vi "testFit.vi"() -> ()   [LabVIEW 2011]
uses:
  <vilib>/Analysis/NI_AALPro.lvlib
panel:
  out "XY Graph":cluster{"Value":dbl[], "Value":dbl[]}[](graph)
  out "Best Exponential Fit":dbl[](array[numeric])
  out "offset 2":dbl=nan
  out "damping":dbl=nan
  out "amplitude":dbl=nan
  in  "amp":dbl=100.0
  in  "alpha":dbl=-0.1
  in  "offset":dbl=20.0
  out "P array":dbl[](array[numeric])
  out "t array":dbl[](array[numeric])
  in  "dt":dbl=1.0
  in  "t":dbl
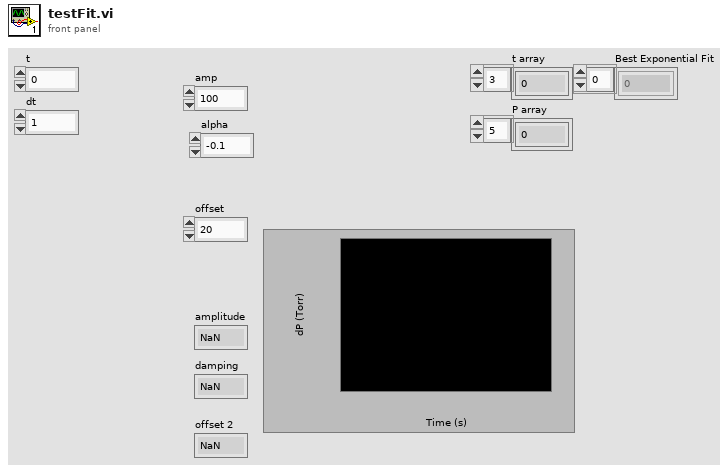
[diagram p1: front panel]
types:
  T1 = cluster{"amp min":dbl, "amp max":dbl, "damping min":dbl, "damping max":dbl, "offset min":dbl, "offset max":dbl}
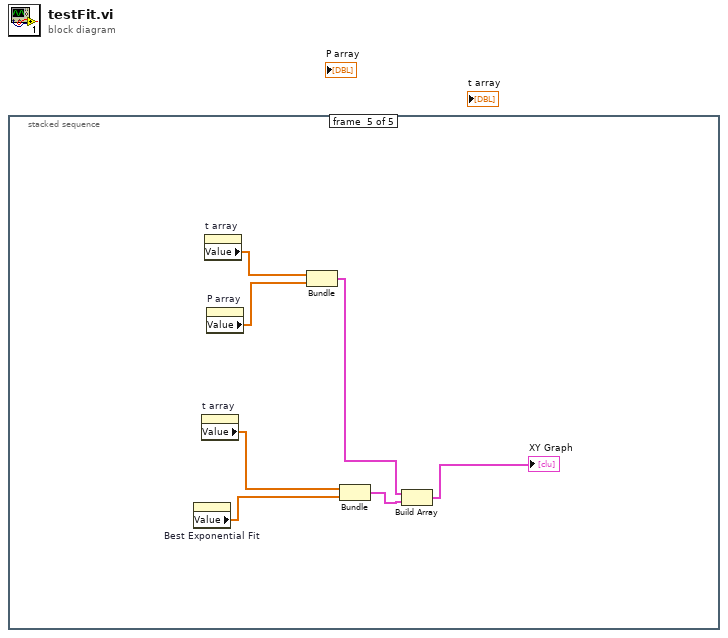
[diagram p0: block diagram]
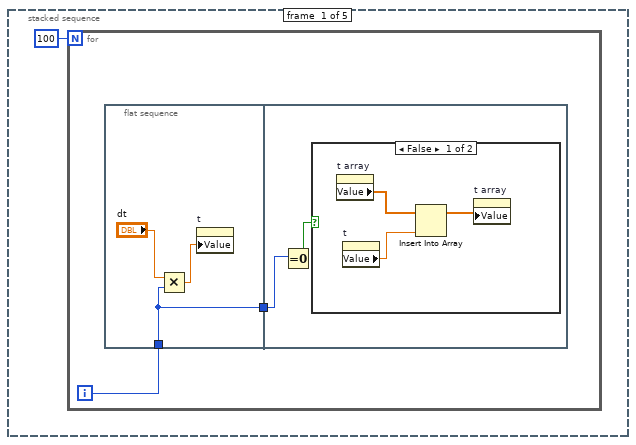
[diagram p2: hidden frame]
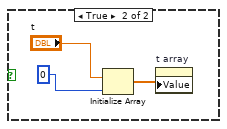
[diagram p3: hidden frame]
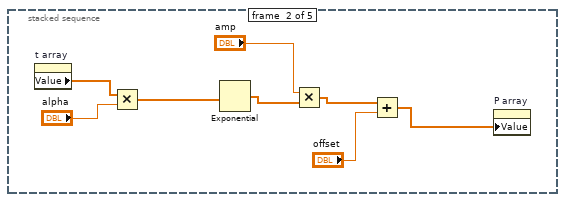
[diagram p4: hidden frame]
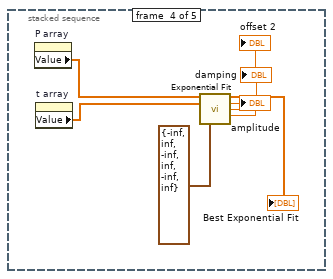
[diagram p6: hidden frame]
diagram:
  n1 = stacked-sequence {
    frame #0 {
      n2 = for {
        N: 100 -> [_]
        i -> [w3]
        n3 = flat-sequence {
          tunnel: w3 -> [w4]
          tunnel: [w4] -> w2
          tunnel: w2 -> [w8]
          frame #0 {
            n4 = Multiply(x="dt", y=w4) -> (x*y=w5:dbl)
            n5 = property on="t" class="DigNum (strict)"("Value"=w5) -> ()  [unwired: 2 in, 2 out]
          }
          frame #1 {
            n6 = Equal To 0?(x=w8) -> (x = 0?=w7:bool)
            n7 = case shown="False" w7 {
              frame False {
                n8 = property on="t array" class="Arr (strict)"() -> ("Value"=w11:dbl[])  [unwired: 2 in, 2 out]
                n9 = property on="t" class="DigNum (strict)"() -> ("Value"=w10:dbl)  [unwired: 2 in, 2 out]
                n10 = Insert Into Array(array=w11, new element=w10) -> (w9:dbl[])  [unwired: 1 in]
                n11 = property on="t array" class="Arr (strict)"("Value"=w9) -> ()  [unwired: 2 in, 2 out]
              }
              frame True {
                n12 = Initialize Array("t", 0 ("dimension size")) -> (w12:dbl[])
                n13 = property on="t array" class="Arr (strict)"("Value"=w12) -> ()  [unwired: 2 in, 2 out]
              }
            }
          }
        }
      }
    }
    frame #1 {
      n14 = property on="t array" class="Arr (strict)"() -> ("Value"=w21:dbl[])  [unwired: 2 in, 2 out]
      n15 = Multiply(x=w21, y="alpha") -> (x*y=w20:dbl[])
      n16 = Exponential(1:w20) -> (0:w17:dbl[])
      n17 = Multiply(x="amp", y=w17) -> (x*y=w16:dbl[])
      n18 = Add(x=w16, y="offset") -> (x+y=w18:dbl[])
      n19 = property on="P array" class="Arr (strict)"("Value"=w18) -> ()  [unwired: 2 in, 2 out]
    }
    frame #2 {
    }
    frame #3 {
      n20 = property on="P array" class="Arr (strict)"() -> ("Value"=w28:dbl[])  [unwired: 2 in, 2 out]
      n21 = property on="t array" class="Arr (strict)"() -> ("Value"=w29:dbl[])  [unwired: 2 in, 2 out]
      n22 = call <vilib>:"Exponential Fit.vi"("Y"=w28, "X"=w29, "parameter bounds"=T1 {"amp min"=-inf, "amp max"=inf, "damping min"=-inf, "damping max"=inf, "offset min"=-inf, "offset max"=inf}) -> ("Best Exponential Fit"=→"Best Exponential Fit":dbl[], "amplitude"=→"amplitude":dbl, "damping"=→"damping":dbl, "offset"=→"offset 2":dbl)  [unwired: 7 in, 2 out]
    }
    frame #4 {
      n23 = property on="Best Exponential Fit" class="Arr (strict)"() -> ("Value"=w35:dbl[])  [unwired: 2 in, 2 out]
      n24 = property on="t array" class="Arr (strict)"() -> ("Value"=w36:dbl[])  [unwired: 2 in, 2 out]
      n25 = property on="t array" class="Arr (strict)"() -> ("Value"=w33:dbl[])  [unwired: 2 in, 2 out]
      n26 = property on="P array" class="Arr (strict)"() -> ("Value"=w32:dbl[])  [unwired: 2 in, 2 out]
      n27 = Bundle("Value"=w33, "Value"=w32) -> (w30:cluster{"Value":dbl[], "Value":dbl[]})  [unwired: 1 in]
      n28 = Bundle("Value"=w36, "Value"=w35) -> (w34:cluster{"Value":dbl[], "Value":dbl[]})  [unwired: 1 in]
      n29 = Build Array "Build Array"(w30, w34) -> (→"XY Graph":cluster{"Value":dbl[], "Value":dbl[]}[])
    }
  }
